vi "Tcp Servers.vi"(7 "Action":T1, 8 "error in (no error)":errorcluster, 9 "VI in":refnum<vi>, 10 "Connection in":refnum<k5>, 11 "Server Port in":u16) -> (0 "error out":errorcluster, 1 "VI out":refnum<vi>, 2 "Connection out":refnum<k5>, 3 "Server Port out":u16)   [LabVIEW 2021, in "HttpServer.lvlib"]
uses:
  HttpServer.lvlib
  TypeDefs/Action.ctl
  <vilib>/Utility/miscctls.llb/LVMapReplaceAction.ctl
  <vilib>/Utility/error.llb/Error Cluster From Error Code.vi
  <vilib>/ErrorRing/Error Ring.xnode
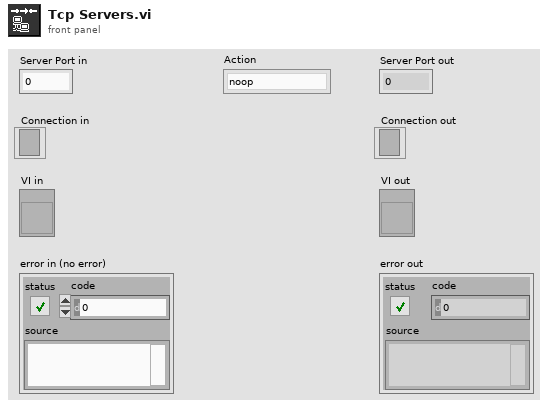
[diagram p1: front panel]
types:
  T1 = typedef "HttpServer.lvlib/Action.ctl" = enum8{"noop", "add", "get", "set", "remove"}
  T2 = map{u16, cluster{"VI":refnum<vi>, "Listener":refnum<k5>}}
  T3 = typedef "LVMapReplaceAction.ctl" = enum32{"Modify Entry only if found", "Add or Modify Entry", "Delete Entry"}
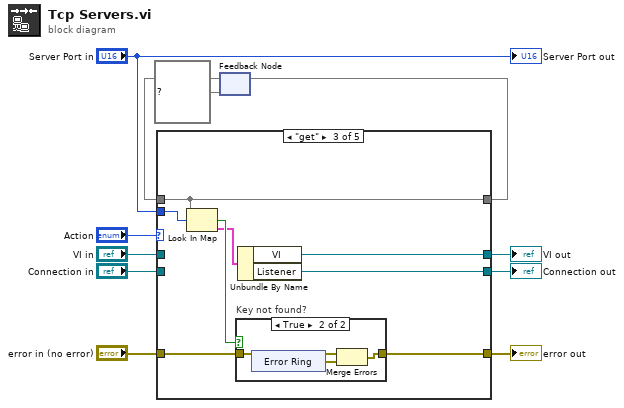
[diagram p0: block diagram]
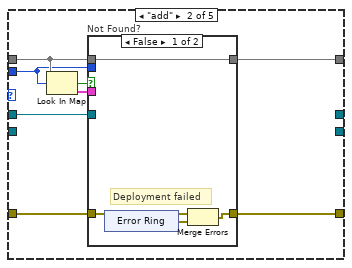
[diagram p3: hidden frame]
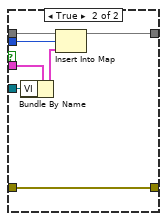
[diagram p4: hidden frame]
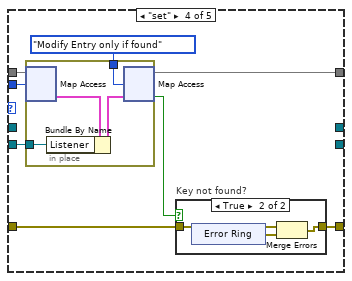
[diagram p6: hidden frame]
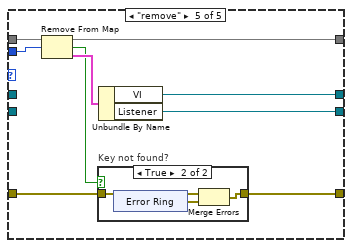
[diagram p8: hidden frame]
diagram:
  n1 = feedback #1(T2 {} ("Servers")) -> (w6:T2)
  n2 = case shown="\"get\"" "Action" {
    tunnel: [w12 w15 w42 w56 w80] -> w10
    tunnel: "error in (no error)" -> [w12 w14 w44 w57 w81]
    tunnel: "Server Port in" -> [_ w17 w40 w58 w75]
    tunnel: w6 -> [w13 w21 w43 w60 w79]
    tunnel: [w13 w20 w43 w53 w78] -> w5
    tunnel: "Connection in" -> [_ _ _ w54 _]
    tunnel: [_ _ w38 _ w74] -> w2
    tunnel: "VI in" -> [_ w16 _ _ _]
    tunnel: [_ _ w37 _ w73] -> w1
    frame "noop" {
    }
    frame "add" {
      n3 = Look In Map(map=w21, key=w17) -> (key not found?=w18:bool, value=w19:cluster{"VI":refnum<vi>, "Listener":refnum<k5>})  [unwired: 1 in]
      n4 = case "Not Found?" shown="False" w18 {
        tunnel: w21 -> [w25 w36]
        tunnel: [w25 w35] -> w20
        tunnel: w19 -> [_ w34]
        tunnel: w17 -> [_ w33]
        tunnel: w16 -> [_ w32]
        tunnel: [w23 w31] -> w15
        tunnel: w14 -> [w24 w31]
        frame False {
          # "Deployment failed"
          n5 = xnode "Error Ring"() -> ("error out"=w22:errorcluster)
          n6 = Merge Errors(w24, w22) -> (w23:errorcluster)
        }
        frame True {
          n7 = Bundle By Name(cluster=w34, "VI"=w32) -> (w30:cluster{"VI":refnum<vi>, "Listener":refnum<k5>})
          n8 = Insert Into Map(map in=w36, key=w33, value=w30) -> (map out=w35:T2)  [unwired: 2 out]
        }
      }
    }
    frame "get" {
      n9 = Look In Map(map=w43, key=w40) -> (key not found?=w41:bool, value=w39:cluster{"VI":refnum<vi>, "Listener":refnum<k5>})  [unwired: 1 in]
      n10 = case "Key not found?" shown="True" w41 {
        tunnel: w44 -> [w45 w48]
        tunnel: [w45 w47] -> w42
        frame False {
        }
        frame True {
          n11 = xnode "Error Ring"() -> ("error out"=w46:errorcluster)
          n12 = Merge Errors(w48, w46) -> (w47:errorcluster)
        }
      }
      n13 = Unbundle By Name(w39) -> ("VI"=w38:refnum<vi>, "Listener"=w37:refnum<k5>)
    }
    frame "set" {
      n14 = in-place {
        in-place-border: LVMapReplaceAction."Modify Entry only if found" ("action") -> [w64]
        in-place-border: w54 -> [w61]
        n15 = in-place-map #2(w60, w58) -> (w63:cluster{"VI":refnum<vi>, "Listener":refnum<k5>})  [unwired: 1 in, 1 out]
        n16 = Bundle By Name(cluster=w63, "Listener"=w61) -> (w62:cluster{"VI":refnum<vi>, "Listener":refnum<k5>})
        n17 = in-place-map #2(w62, w64) -> (w53:T2, w55:bool)  [unwired: 1 out]
      }
      n18 = case "Key not found?" shown="True" w55 {
        tunnel: w57 -> [w65 w68]
        tunnel: [w65 w67] -> w56
        frame False {
        }
        frame True {
          n19 = xnode "Error Ring"() -> ("error out"=w66:errorcluster)
          n20 = Merge Errors(w68, w66) -> (w67:errorcluster)
        }
      }
    }
    frame "remove" {
      n21 = Remove From Map(10:w75, 11:w79) -> (1:w77:cluster{"VI":refnum<vi>, "Listener":refnum<k5>}, 2:w76:bool, 3:w78:T2)
      n22 = case "Key not found?" shown="True" w76 {
        tunnel: w81 -> [w82 w85]
        tunnel: [w82 w84] -> w80
        frame False {
        }
        frame True {
          n23 = xnode "Error Ring"() -> ("error out"=w83:errorcluster)
          n24 = Merge Errors(w85, w83) -> (w84:errorcluster)
        }
      }
      n25 = Unbundle By Name(w77) -> ("VI"=w74:refnum<vi>, "Listener"=w73:refnum<k5>)
    }
  }
  "error out" <- w10
  "VI out" <- w2
  "Connection out" <- w1
  n26 = feedback-in #1(w5) -> ()
  "Server Port out" <- "Server Port in"
